vi "ROI entry- extract Z start and stop from motor Z.vi"(8 "error in (no error)":errorcluster, 10 "Z Plane Idx":i32[](array[numeric]), 11 "Z motor planes":dbl[](array[numeric])) -> (0 "error out":errorcluster, 1 "No of Lines":i32, 2 "Z stop(m)":dbl, 3 "Z start(m)":dbl)   [LabVIEW 2020]
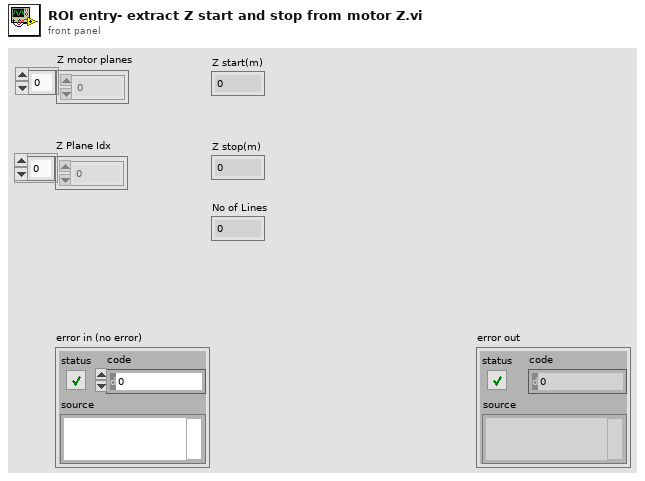
[diagram p1: front panel]
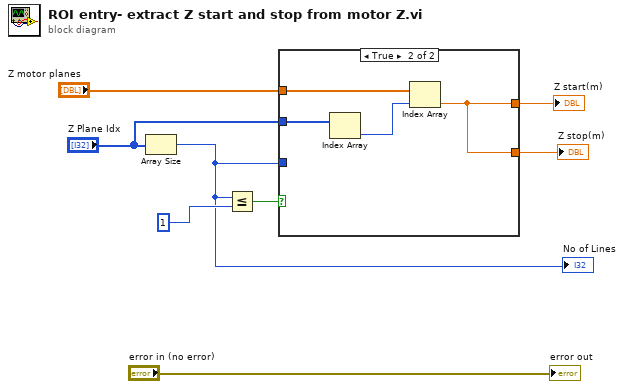
[diagram p0: block diagram]
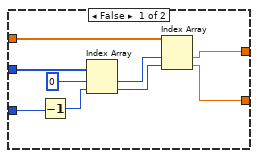
[diagram p2: hidden frame]
diagram:
  n1 = Array Size(array="Z Plane Idx") -> (size(s)=w4:i32)
  "No of Lines" <- w4
  n2 = Less Or Equal?(x=w4, y=1) -> (x <= y?=w3:bool)
  n3 = case shown="True" w3 {
    tunnel: "Z motor planes" -> [w17 w21]
    tunnel: [w14 w18] -> w6
    tunnel: "Z Plane Idx" -> [w16 w20]
    tunnel: w4 -> [w12 _]
    tunnel: [w9 w18] -> w2
    frame False {
      n4 = Decrement(x=w12) -> (x-1=w11:i32)
      n5 = Index Array(array=w16, index #1=0 ("index"), index #2=w11) -> (element #1=w15:i32, element #2=w10:i32)
      n6 = Index Array(array=w17, index #1=w15, index #2=w10) -> (element #1=w14:dbl, element #2=w9:dbl)
    }
    frame True {
      n7 = Index Array(array=w20) -> (element=w19:i32)  [unwired: 1 in]
      n8 = Index Array(array=w21, index=w19) -> (element=w18:dbl)
    }
  }
  "Z start(m)" <- w6
  "Z stop(m)" <- w2
  "error out" <- "error in (no error)"
